vi "write_DAC_word.vi"(10 "U16 data number":u16, 11 "DAC values in":T1 {"bit index" min=-1 max=17 step=1; "channel index" max=7 step=1; "offset" max=4095; "DAC voltage"."ch1" max=4095 step=1; "DAC voltage"."ch0" max=4095 step=1}) -> (3 "DAC values out":T1 {"bit index" min=-1 max=17 step=1; "channel index" max=7 step=1; "offset" max=4095; "DAC voltage"."ch1" max=4095 step=1; "DAC voltage"."ch0" max=4095 step=1})   [LabVIEW 2011]
uses:
  typedefs/DAC_values_cluster.ctl
  typedefs/DAC_voltage_cluster.ctl
  <vilib>/rvi/eio/common/nirviEmuTemplateMethod_errors.vi
  <vilib>/eio/EIONode/EIONode.xnode
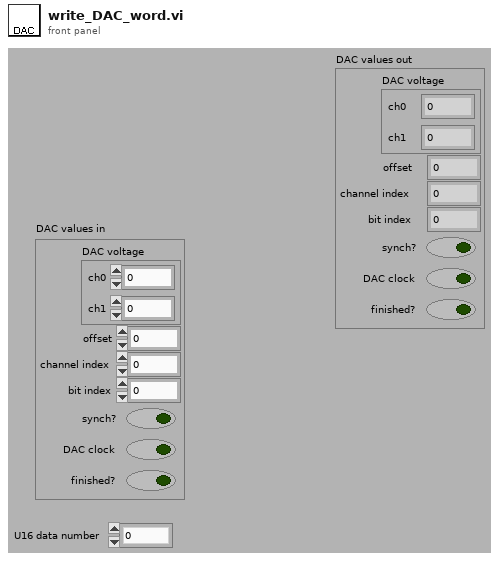
[diagram p1: front panel]
types:
  T1 = typedef "DAC_values_cluster.ctl" = cluster{"DAC voltage":T2, "offset":u16, "channel index":u16, "bit index":i32, "synch?":bool, "DAC clock":bool, "finished?":bool}
  T2 = typedef "DAC_voltage_cluster.ctl" = cluster{"ch0":u16, "ch1":u16}
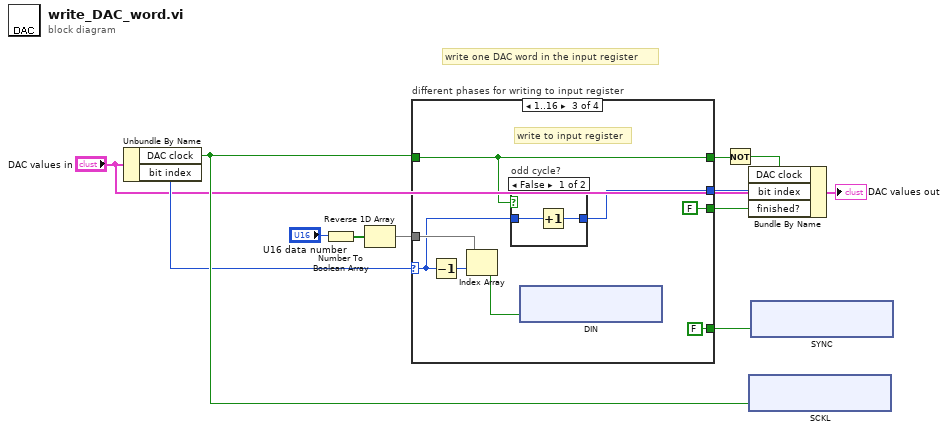
[diagram p0: block diagram]
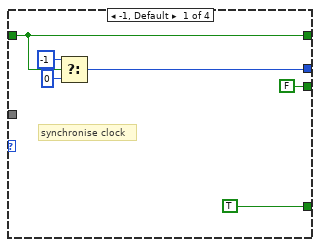
[diagram p2: hidden frame]
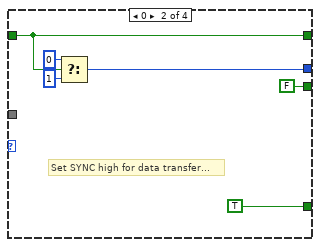
[diagram p3: hidden frame]
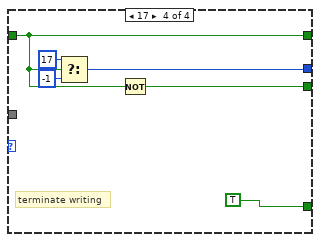
[diagram p5: hidden frame]
diagram:
  # "write one DAC word in the input register"
  n1 = Unbundle By Name("DAC values in") -> ("DAC clock"=w7:bool, "bit index"=w6:i32)
  n2 = Number To Boolean Array(number="U16 data number") -> (Boolean array=w12:bool[])
  n3 = Reverse 1D Array(array=w12) -> (reversed array=w10:bool[])
  n4 = case "different phases for writing to input register" shown="1..16" w6 {
    selector: w6 -> [_ _ w25 _]
    tunnel: w7 -> [w16 w20 w30 w37]
    tunnel: [w15 w22 w29 w39] -> w3
    tunnel: [TRUE ("SYNC") TRUE ("SYNC") FALSE ("SYNC") TRUE ("SYNC")] -> w8
    tunnel: w10 -> [_ _ w31 _]
    tunnel: [w16 w20 w30 w37] -> w9
    tunnel: [FALSE FALSE FALSE w36] -> w2
    frame -1, Default {
      # "synchronise clock"
      n5 = Select(t=-1, s=w16, f=0) -> (s? t:f=w15:i32)
    }
    frame 0 {
      # "Set SYNC high for data transfer..."
      n6 = Select(t=0, s=w20, f=1) -> (s? t:f=w22:i32)
    }
    frame 1..16 {
      # "write to input register"
      n7 = Decrement(x=w25) -> (x-1=w32:i32)
      n8 = Index Array(array=w31, index=w32) -> (element=w27:bool)
      n9 = case "odd cycle?" shown="False" w30 {
        tunnel: w25 -> [w33 w35]
        tunnel: [w34 w35] -> w29
        frame False {
          n10 = Increment(x=w33) -> (x+1=w34:i32)
        }
        frame True {
        }
      }
      n11 = xnode "DIN"("Connector1/DIO36"=w27) -> ()  [unwired: 1 in, 1 out]
    }
    frame 17 {
      # "terminate writing"
      n12 = Select(t=17, s=w37, f=-1) -> (s? t:f=w39:i32)
      n13 = Not(x=w37) -> (.not. x?=w36:bool)
    }
  }
  n14 = Not(x=w9) -> (.not. x?=w4:bool)
  n15 = Bundle By Name(cluster="DAC values in", "DAC clock"=w4, "bit index"=w3, "finished?"=w2) -> (→"DAC values out":T1)
  n16 = xnode "SCKL"("Connector1/DIO38"=w7) -> ()  [unwired: 1 in, 1 out]
  n17 = xnode "SYNC"("Connector1/DIO34"=w8) -> ()  [unwired: 1 in, 1 out]
